vi "SussRegisterProberApp.vi"(2 "error in (no error)":errorcluster, 3 "Flag":i32(ring) items=["Disabled, Multiple App", "Enabled, Single App", "Disabled, Single App"], 4 "AppName":string="LabVIEW", 5 "Groupname":string="LabVIEW") -> (0 "error out":errorcluster, 1 "RegistrationNumber":T1)   [LabVIEW 2012]
doc: "RegisterProberApp\n\nAny application that will communicate with ProberBench must first call this function to register itself with the Message Server. The application must make a corresponging call to CloseProberApp() before it closes. AppName provides a text description of the application to be used in data logging, for instance by the MsgWin.exe utility. GroupName is significant only in the unusual case where your application will handle the commands in a ProberBench command-group (requiring it to poll GetCommand()); in this case, GroupName must match the target command-group name as found in commands.txt. Generally, you can pass the same string for both AppName and GroupName. The Flag parameter bit 0 determines whether the ProberBench Server will send notifications to the application (bit 0 set enables notifications). The Flag parameter bit 1 determines whether only one application can be registered with this name (bit 1 set allows only one application with this name to be registered). Return value is a positive registration number if successful, or zero on failure.\n\nInput: AppName, GroupName, Flag\nOutput: RegistrationNumber\nReturns: Greater than zero upon success\n\n\n\nCopyright © 2001 Karl Suss Dresden GmbH, All Rights Reserved."
uses:
  <instrlib>/SUSSProberInterface/SussProberInterface.llb/RegistrationNumber.ctl
  msgserve.dll
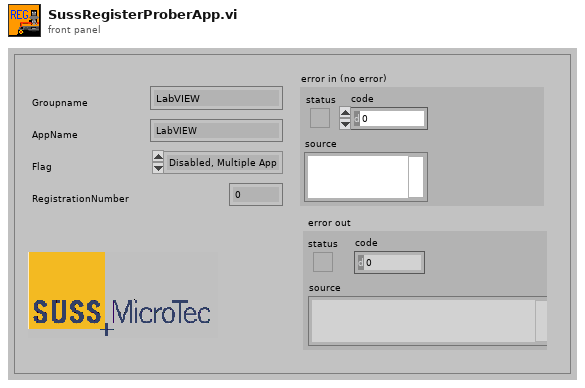
[diagram p1: front panel]
types:
  T1 = typedef "RegistrationNumber.ctl" = i32
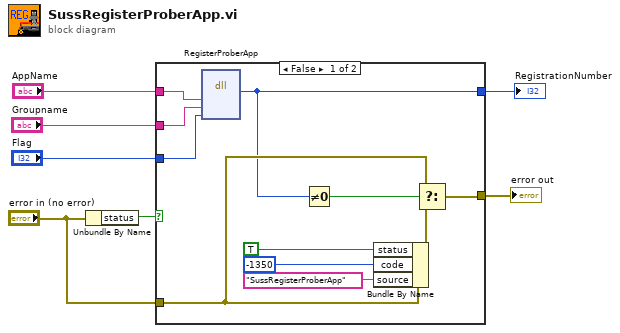
[diagram p0: block diagram]
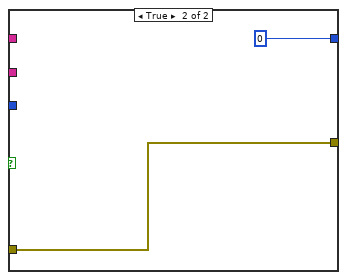
[diagram p2: hidden frame]
diagram:
  n1 = Unbundle By Name("error in (no error)") -> ("status"=w7:bool)
  n2 = case shown="False" w7 {
    tunnel: "error in (no error)" -> [w15 w20]
    tunnel: [w13 w20] -> w5
    tunnel: "AppName" -> [w12 _]
    tunnel: "Groupname" -> [w11 _]
    tunnel: "Flag" -> [w10 _]
    tunnel: [w8 0] -> w1
    frame False {
      n3 = dll-call lib="msgserve.dll" fn="RegisterProberApp"("AppName"=w12, "ClassName"=w11, "Notify"=w10) -> (w8:i32)  [unwired: 6 in, 2 out]
      n4 = Not Equal To 0?(x=w8) -> (x != 0?=w9:bool)
      n5 = Bundle By Name(cluster=w15, "status"=TRUE ("Bundle Element"), "code"=-1350 ("Bundle Element"), "source"="SussRegisterProberApp" ("Bundle Element")) -> (w14:errorcluster)
      n6 = Select(t=w15, s=w9, f=w14) -> (s? t:f=w13:errorcluster)
    }
    frame True {
    }
  }
  "error out" <- w5
  "RegistrationNumber" <- w1
